vi "Launching Actor.vi"(7 "Auto Dispose Ref":bool, 8 "error in (no error)":errorcluster, 9 "Root Actor Address":refnum<class "Mail Strategy.lvclass">, 11 "System Actor in":refnum<class "System Actor.lvclass">) -> (0 "error out":errorcluster, 2 "VI Refnum":refnum<vi>, 3 "System Actor out":refnum<class "System Actor.lvclass">)   [LabVIEW 2024, in "System Actor.lvclass"]
uses:
  System Actor.lvclass
  Messenger/Mail Strategy/Mail Strategy.lvclass
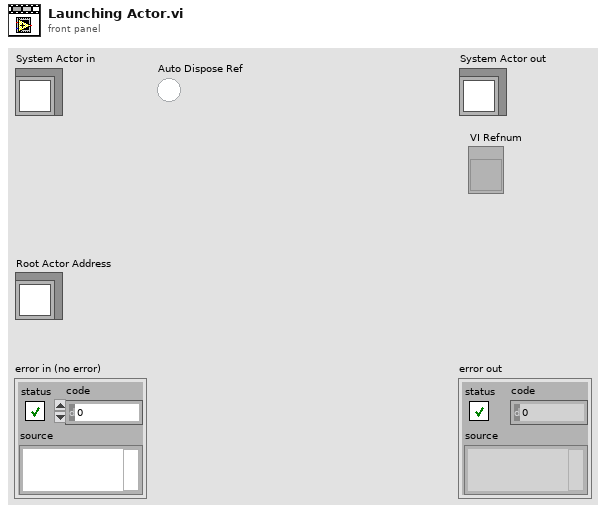
[diagram p1: front panel]
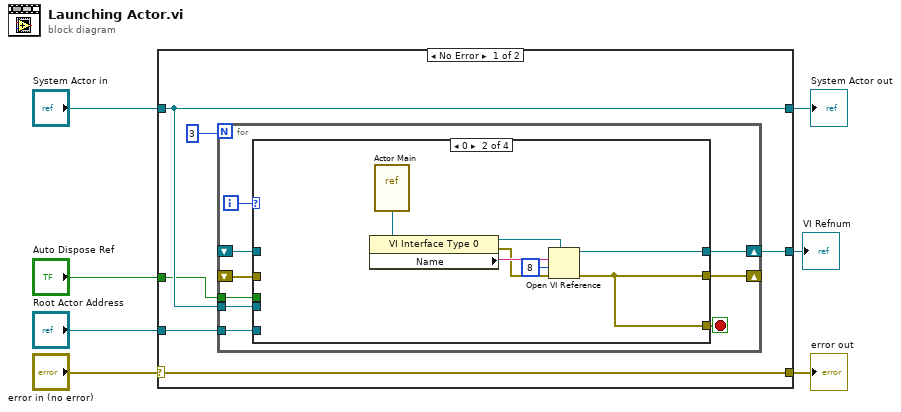
[diagram p0: block diagram]
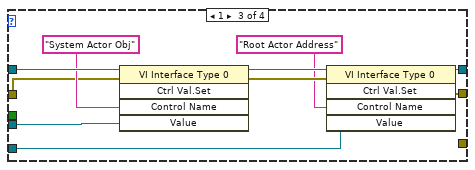
[diagram p3: hidden frame]
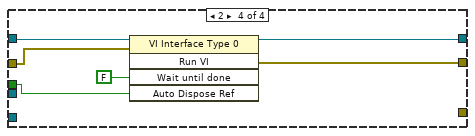
[diagram p4: hidden frame]
diagram:
  n1 = case shown="No Error" "error in (no error)" {
    selector: "error in (no error)" -> [w13 w49]
    tunnel: [w13 w49] -> w6
    tunnel: [w11 w48] -> w4
    tunnel: "System Actor in" -> [w11 w48]
    tunnel: [w10 _] -> w3
    tunnel: "Root Actor Address" -> [w9 _]
    tunnel: "Auto Dispose Ref" -> [w8 _]
    frame No Error {
      n2 = for {
        N: 3 -> [_]
        tunnel: w11 -> [w21]
        shift-right: [w19] -> w10
        shift-left: _ -> [w18]
        shift-right: [w17] -> _
        shift-left: _ -> [w16]
        tunnel: w9 -> [w15]
        tunnel: w8 -> [w14]
        i -> [w22]
        stop <- w20 stop-if-true
        n3 = case shown="0" w22 {
          tunnel: w21 -> [_ _ w40 _]
          tunnel: [_ w25 _ _] -> w20
          tunnel: [w24 w26 w37 w44] -> w19
          tunnel: w18 -> [w24 _ w41 w46]
          tunnel: [w23 w25 w36 w43] -> w17
          tunnel: w16 -> [w23 _ w38 w45]
          tunnel: w15 -> [_ _ w33 _]
          tunnel: w14 -> [_ _ _ w42]
          frame -1, Default {
          }
          frame 0 {
            n4 = vi-ref "Actor Main.vi"() -> (w31:refnum<vi>)
            n5 = property class="VI Interface Type 0"(reference=w31) -> (reference out=w30:refnum<vi>, error out=w28:errorcluster, "Name"=w29:string)  [unwired: 1 in]
            n6 = Open VI Reference(type specifier VI Refnum (for type only)=w30, vi path=w29, options=8, error in (no error)=w28) -> (vi reference=w26:refnum<vi>, error out=w25:errorcluster)  [unwired: 2 in]
          }
          frame 1 {
            n7 = invoke class="VI Interface Type 0" method="Ctrl Val.Set"(reference=w41, error in=w38, "Control Name"="System Actor Obj", "Value"=w40) -> (reference out=w35:refnum<vi>, error out=w34:errorcluster)  [unwired: 1 in, 3 out]
            n8 = invoke class="VI Interface Type 0" method="Ctrl Val.Set"(reference=w35, error in=w34, "Control Name"="Root Actor Address", "Value"=w33) -> (reference out=w37:refnum<vi>, error out=w36:errorcluster)  [unwired: 1 in, 3 out]
          }
          frame 2 {
            n9 = invoke class="VI Interface Type 0" method="Run VI"(reference=w46, error in=w45, "Wait until done"=FALSE ("Wait Until Done"), "Auto Dispose Ref"=w42) -> (reference out=w44:refnum<vi>, error out=w43:errorcluster)  [unwired: 1 in, 3 out]
          }
        }
      }
    }
    frame Error {
    }
  }
  "error out" <- w6
  "System Actor out" <- w4
  "VI Refnum" <- w3
